vi "Teleop.vi"(10 "Match Info":T1={"Autonomous Elapsed Seconds"=0.0, "TeleOp Elapsed Seconds"=0.0, "Disabled Elapsed Seconds"=0.0, "Visited Autonomous"=FALSE, "Visited TeleOp"=FALSE, "Visited Disabled"=FALSE, "Autonomous Settings"={"Autonomous Style"=enum."Independent", "VI Refnum"=refnum}}, 11 "Call Context":T2) -> ()   [LabVIEW 2012]
doc: "This VI is called for each TeleOp packet received from the DS where the robot is not disabled. It is often used to read from the joysticks and update I/O or to update setpoints for timed control loops. It should complete and return within 20 milliseconds or it may miss DS packets."
uses:
  <vilib>/Rock Robotics/WPI/DriverStation/WPI_DriverStationDerivedRobotMode.ctl
  <vilib>/Rock Robotics/WPI/DriverStation/WPI_DriverStationMatch Info.ctl
  Sidestep Globals.vi
  Robot Global Data.vi
  <vilib>/Rock Robotics/Network Tables/SD Write Number.vi
  <vilib>/Rock Robotics/Network Tables/SD Write String.vi
  <vilib>/Rock Robotics/Network Tables/SD Write Boolean.vi
panel:
  in  "Hotkey Timer":dbl
  in  "Hotkey Step":i16
  out "Hotkey Running?":bool
  in  "Current Hotkey":string
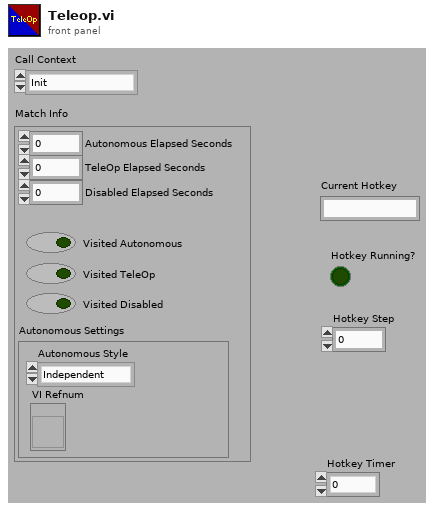
[diagram p1: front panel]
types:
  T1 = typedef "WPI_DriverStationMatch Info.ctl" = cluster{"Autonomous Elapsed Seconds":dbl, "TeleOp Elapsed Seconds":dbl, "Disabled Elapsed Seconds":dbl, "Visited Autonomous":bool, "Visited TeleOp":bool, "Visited Disabled":bool, "Autonomous Settings":cluster{"Autonomous Style":enum16{"Iterative", "Independent"}, "VI Refnum":refnum<vi>}}
  T2 = typedef "WPI_DriverStationDerivedRobotMode.ctl" = enum16{"Init", "Execute", "Stop"}
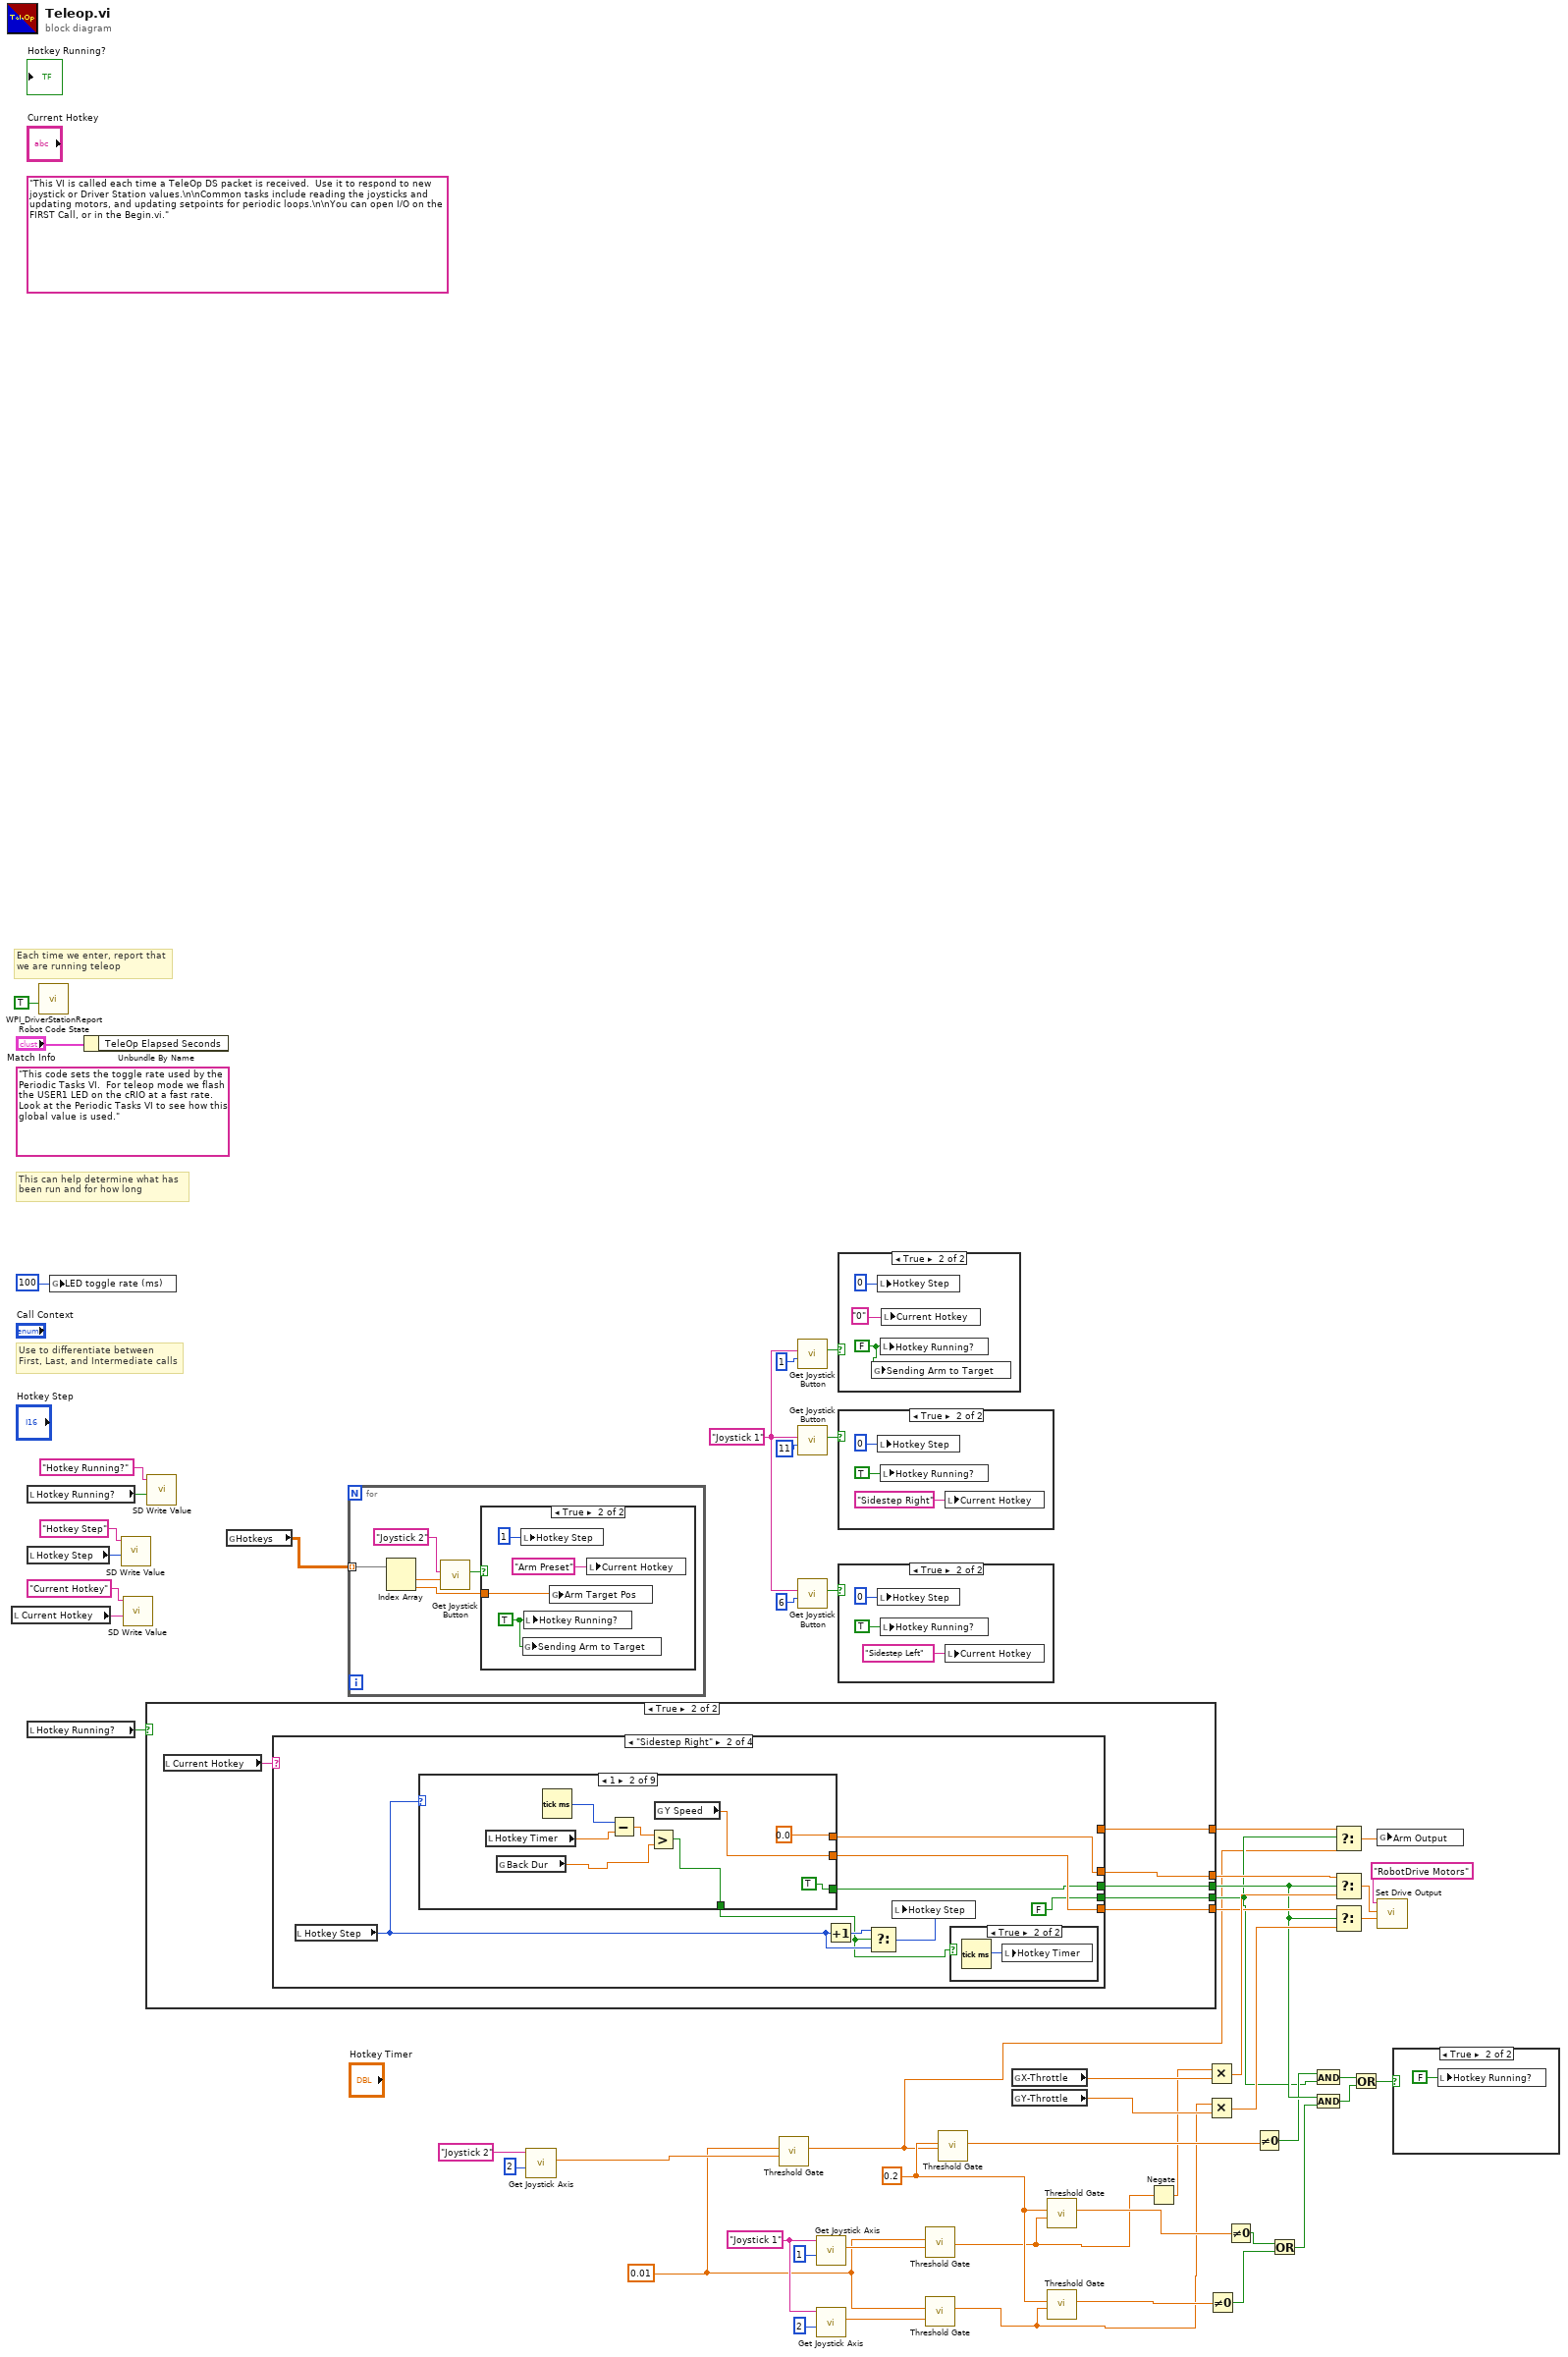
[diagram p0: block diagram]
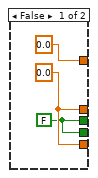
[diagram p5: hidden frame]
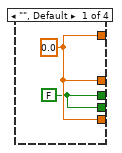
[diagram p6: hidden frame]
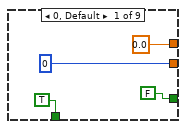
[diagram p8: hidden frame]
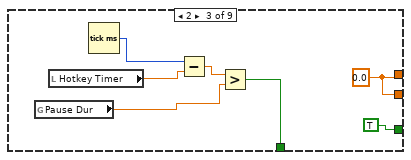
[diagram p9: hidden frame]
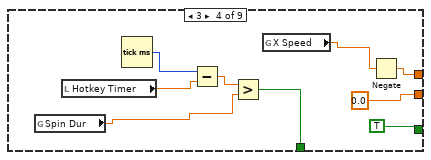
[diagram p10: hidden frame]
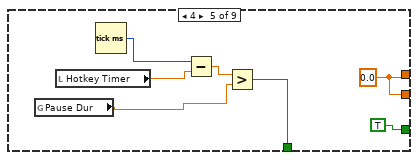
[diagram p11: hidden frame]
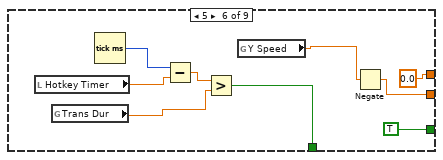
[diagram p12: hidden frame]
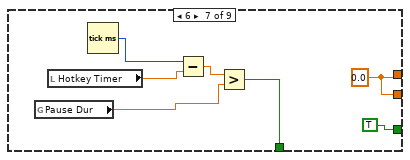
[diagram p13: hidden frame]
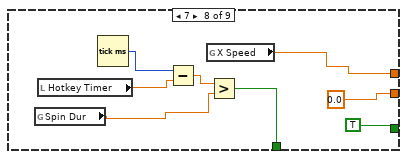
[diagram p14: hidden frame]
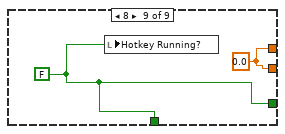
[diagram p15: hidden frame]
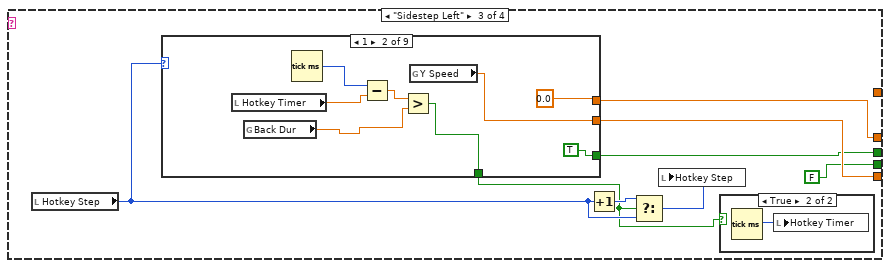
[diagram p16: hidden frame]
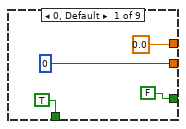
[diagram p18: hidden frame]
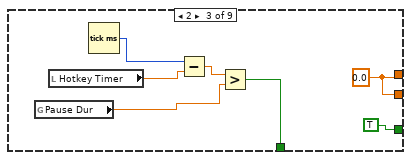
[diagram p19: hidden frame]
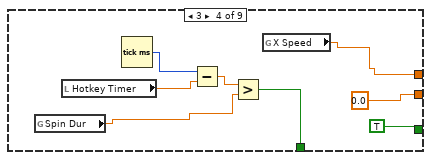
[diagram p20: hidden frame]
diagram:
  w9 = "Joystick 1"
  w30 = 0.2
  w48 = "Joystick 1"
  w13 = 0.01
  (unwired) "This code sets the toggle rate used by the Periodic Tasks VI.  For teleop mode we flash the USER1 LED on the cRIO at a fast rate.  Look at the Periodic Tasks VI to see how this global value is used."
  (unwired) "This VI is called each time a TeleOp DS packet is received.  Use it to respond to new joystick or Driver Station values.\n\nCommon tasks include reading the joysticks and updating motors, and updating setpoints for periodic loops.\n\nYou can open I/O on the FIRST Call, or in the Begin.vi."
  # "Each time we enter, report that\nwe are running teleop"
  # "Use to differentiate between\nFirst, Last, and Intermediate calls"
  # "This can help determine what has\nbeen run and for how long"
  n1 = local read "Current Hotkey"() -> (w27:string)
  n2 = local read "Hotkey Running?"() -> (w29:bool)
  n3 = local read "Hotkey Step"() -> (w28:i16)
  n4 = local read "Hotkey Running?"() -> (w40:bool)
  n5 = call <vilib>:"WPI_DriverStationReport Robot Code State.vi"("TeleOp"=TRUE ("Autonomous")) -> ()  [unwired: 10 in, 1 out]
  n6 = global write "Robot Global Data.vi" "LED toggle rate (ms)"(u32 100 ("LED ms toggle rate")) -> ()
  n7 = Unbundle By Name("Match Info") -> ()  [unwired: 1 out]
  n8 = call-poly <vilib>:"SD Write Value.vi"("Numeric"=w28, "Name"="Hotkey Step") -> ()  [unwired: 8 in, 2 out]
  n9 = call-poly <vilib>:"SD Write Value.vi"("String"=w27, "Name"="Current Hotkey") -> ()  [unwired: 8 in, 2 out]
  n10 = case shown="True" w40 {
    tunnel: [0.0 w63] -> w39
    tunnel: [w56 w62] -> w18
    tunnel: [w57 w60] -> w34
    tunnel: [w57 w61] -> w31
    tunnel: [w56 w59] -> w20
    frame False {
      w57 = 0.0
      w56 = FALSE
    }
    frame True {
      n11 = local read "Current Hotkey"() -> (w64:string)
      n12 = case shown="\"Sidestep Right\"" w64 {
        tunnel: [w66 _ _ w210] -> w63
        tunnel: [w65 FALSE FALSE w209] -> w62
        tunnel: [w66 w71 w141 w208] -> w61
        tunnel: [w66 w67 w137 w208] -> w60
        tunnel: [w65 w70 w140 FALSE] -> w59
        frame "", Default {
          w65 = FALSE
          w66 = 0.0
        }
        frame "Sidestep Right" {
          n13 = local read "Hotkey Step"() -> (w72:i16)
          n14 = case shown="1" w72 {
            tunnel: [TRUE w83 w90 w100 w106 w116 w122 w131 w136] -> w68
            tunnel: [0 w80 w94 0.0 w110 w111 w126 0.0 w135] -> w71
            tunnel: [FALSE TRUE TRUE TRUE TRUE TRUE TRUE TRUE w136] -> w70
            tunnel: [0.0 0.0 w94 w97 w110 0.0 w126 w127 w135] -> w67
            frame 0, Default {
            }
            frame 1 {
              n15 = local read "Hotkey Timer"() -> (w85:dbl)
              n16 = global read "Sidestep Globals.vi" "Back Dur"() -> (w81:dbl)
              n17 = Tick Count (ms)() -> (millisecond timer value=w86:u32)
              n18 = Subtract(x=w86, y=w85) -> (x-y=w84:dbl)
              n19 = Greater?(x=w84, y=w81) -> (0:w83:bool)
              n20 = global read "Sidestep Globals.vi" "Y Speed"() -> (w80:dbl)
            }
            frame 2 {
              w94 = 0.0
              n21 = global read "Sidestep Globals.vi" "Pause Dur"() -> (w88:dbl)
              n22 = local read "Hotkey Timer"() -> (w93:dbl)
              n23 = Tick Count (ms)() -> (millisecond timer value=w91:u32)
              n24 = Subtract(x=w91, y=w93) -> (x-y=w92:dbl)
              n25 = Greater?(x=w92, y=w88) -> (0:w90:bool)
            }
            frame 3 {
              n26 = global read "Sidestep Globals.vi" "Spin Dur"() -> (w96:dbl)
              n27 = local read "Hotkey Timer"() -> (w103:dbl)
              n28 = Tick Count (ms)() -> (millisecond timer value=w101:u32)
              n29 = Subtract(x=w101, y=w103) -> (x-y=w102:dbl)
              n30 = Greater?(x=w102, y=w96) -> (0:w100:bool)
              n31 = global read "Sidestep Globals.vi" "X Speed"() -> (w95:dbl)
              n32 = Negate(x=w95) -> (-x=w97:dbl)
            }
            frame 4 {
              w110 = 0.0
              n33 = global read "Sidestep Globals.vi" "Pause Dur"() -> (w104:dbl)
              n34 = local read "Hotkey Timer"() -> (w109:dbl)
              n35 = Tick Count (ms)() -> (millisecond timer value=w107:u32)
              n36 = Subtract(x=w107, y=w109) -> (x-y=w108:dbl)
              n37 = Greater?(x=w108, y=w104) -> (0:w106:bool)
            }
            frame 5 {
              n38 = local read "Hotkey Timer"() -> (w118:dbl)
              n39 = global read "Sidestep Globals.vi" "Trans Dur"() -> (w113:dbl)
              n40 = Tick Count (ms)() -> (millisecond timer value=w119:u32)
              n41 = Subtract(x=w119, y=w118) -> (x-y=w117:dbl)
              n42 = Greater?(x=w117, y=w113) -> (0:w116:bool)
              n43 = global read "Sidestep Globals.vi" "Y Speed"() -> (w112:dbl)
              n44 = Negate(x=w112) -> (-x=w111:dbl)
            }
            frame 6 {
              w126 = 0.0
              n45 = global read "Sidestep Globals.vi" "Pause Dur"() -> (w120:dbl)
              n46 = local read "Hotkey Timer"() -> (w125:dbl)
              n47 = Tick Count (ms)() -> (millisecond timer value=w123:u32)
              n48 = Subtract(x=w123, y=w125) -> (x-y=w124:dbl)
              n49 = Greater?(x=w124, y=w120) -> (0:w122:bool)
            }
            frame 7 {
              n50 = global read "Sidestep Globals.vi" "Spin Dur"() -> (w128:dbl)
              n51 = local read "Hotkey Timer"() -> (w134:dbl)
              n52 = Tick Count (ms)() -> (millisecond timer value=w132:u32)
              n53 = Subtract(x=w132, y=w134) -> (x-y=w133:dbl)
              n54 = global read "Sidestep Globals.vi" "X Speed"() -> (w127:dbl)
              n55 = Greater?(x=w133, y=w128) -> (0:w131:bool)
            }
            frame 8 {
              w135 = 0.0
              w136 = FALSE
              n56 = local write "Hotkey Running?"(w136) -> ()
            }
          }
          n57 = Increment(x=w72) -> (x+1=w74:i16)
          n58 = Select(t=w74, s=w68, f=w72) -> (s? t:f=w73:i16)
          n59 = local write "Hotkey Step"(w73) -> ()
          n60 = case shown="True" w68 {
            frame False {
            }
            frame True {
              n61 = Tick Count (ms)() -> (millisecond timer value=w75:u32)
              n62 = local write "Hotkey Timer"(w75) -> ()
            }
          }
        }
        frame "Sidestep Left" {
          n63 = local read "Hotkey Step"() -> (w142:i16)
          n64 = case shown="1" w142 {
            tunnel: [TRUE w153 w160 w169 w175 w185 w191 w201 w206] -> w138
            tunnel: [0 w150 w164 0.0 w179 w181 w195 0.0 w205] -> w141
            tunnel: [FALSE TRUE TRUE TRUE TRUE TRUE TRUE TRUE w206] -> w140
            tunnel: [0.0 0.0 w164 w165 w179 0.0 w195 w196 w205] -> w137
            frame 0, Default {
            }
            frame 1 {
              n65 = local read "Hotkey Timer"() -> (w155:dbl)
              n66 = global read "Sidestep Globals.vi" "Back Dur"() -> (w151:dbl)
              n67 = Tick Count (ms)() -> (millisecond timer value=w156:u32)
              n68 = Subtract(x=w156, y=w155) -> (x-y=w154:dbl)
              n69 = Greater?(x=w154, y=w151) -> (0:w153:bool)
              n70 = global read "Sidestep Globals.vi" "Y Speed"() -> (w150:dbl)
            }
            frame 2 {
              w164 = 0.0
              n71 = global read "Sidestep Globals.vi" "Pause Dur"() -> (w158:dbl)
              n72 = local read "Hotkey Timer"() -> (w163:dbl)
              n73 = Tick Count (ms)() -> (millisecond timer value=w161:u32)
              n74 = Subtract(x=w161, y=w163) -> (x-y=w162:dbl)
              n75 = Greater?(x=w162, y=w158) -> (0:w160:bool)
            }
            frame 3 {
              n76 = global read "Sidestep Globals.vi" "Spin Dur"() -> (w166:dbl)
              n77 = local read "Hotkey Timer"() -> (w172:dbl)
              n78 = Tick Count (ms)() -> (millisecond timer value=w170:u32)
              n79 = Subtract(x=w170, y=w172) -> (x-y=w171:dbl)
              n80 = Greater?(x=w171, y=w166) -> (0:w169:bool)
              n81 = global read "Sidestep Globals.vi" "X Speed"() -> (w165:dbl)
            }
            frame 4 {
              w179 = 0.0
              n82 = global read "Sidestep Globals.vi" "Pause Dur"() -> (w173:dbl)
              n83 = local read "Hotkey Timer"() -> (w178:dbl)
              n84 = Tick Count (ms)() -> (millisecond timer value=w176:u32)
              n85 = Subtract(x=w176, y=w178) -> (x-y=w177:dbl)
              n86 = Greater?(x=w177, y=w173) -> (0:w175:bool)
            }
            frame 5 {
              n87 = local read "Hotkey Timer"() -> (w187:dbl)
              n88 = global read "Sidestep Globals.vi" "Trans Dur"() -> (w182:dbl)
              n89 = Tick Count (ms)() -> (millisecond timer value=w188:u32)
              n90 = Subtract(x=w188, y=w187) -> (x-y=w186:dbl)
              n91 = Greater?(x=w186, y=w182) -> (0:w185:bool)
              n92 = global read "Sidestep Globals.vi" "Y Speed"() -> (w180:dbl)
              n93 = Negate(x=w180) -> (-x=w181:dbl)
            }
            frame 6 {
              w195 = 0.0
              n94 = global read "Sidestep Globals.vi" "Pause Dur"() -> (w189:dbl)
              n95 = local read "Hotkey Timer"() -> (w194:dbl)
              n96 = Tick Count (ms)() -> (millisecond timer value=w192:u32)
              n97 = Subtract(x=w192, y=w194) -> (x-y=w193:dbl)
              n98 = Greater?(x=w193, y=w189) -> (0:w191:bool)
            }
            frame 7 {
              n99 = global read "Sidestep Globals.vi" "Spin Dur"() -> (w199:dbl)
              n100 = local read "Hotkey Timer"() -> (w204:dbl)
              n101 = Tick Count (ms)() -> (millisecond timer value=w202:u32)
              n102 = Subtract(x=w202, y=w204) -> (x-y=w203:dbl)
              n103 = global read "Sidestep Globals.vi" "X Speed"() -> (w197:dbl)
              n104 = Greater?(x=w203, y=w199) -> (0:w201:bool)
              n105 = Negate(x=w197) -> (-x=w196:dbl)
            }
            frame 8 {
              w205 = 0.0
              w206 = FALSE
              n106 = local write "Hotkey Running?"(w206) -> ()
            }
          }
          n107 = Increment(x=w142) -> (x+1=w144:i16)
          n108 = Select(t=w144, s=w138, f=w142) -> (s? t:f=w143:i16)
          n109 = local write "Hotkey Step"(w143) -> ()
          n110 = case shown="True" w138 {
            frame False {
            }
            frame True {
              n111 = Tick Count (ms)() -> (millisecond timer value=w145:u32)
              n112 = local write "Hotkey Timer"(w145) -> ()
            }
          }
        }
        frame "Arm Preset" {
          w208 = 0.0
          n113 = local read "Hotkey Step"() -> (w213:i16)
          n114 = case shown="2" w213 {
            tunnel: [w215 w218] -> w214
            tunnel: [_ 0.0] -> w210
            tunnel: [FALSE w218] -> w209
            frame 1, Default {
              n115 = global read "Robot Global Data.vi" "Sending Arm to Target"() -> (w217:bool)
              n116 = Not(x=w217) -> (.not. x?=w215:bool)
            }
            frame 2 {
              w218 = FALSE
            }
          }
          n117 = Increment(x=w213) -> (x+1=w212:i16)
          n118 = Select(t=w212, s=w214, f=w213) -> (s? t:f=w211:i16)
          n119 = local write "Hotkey Step"(w211) -> ()
        }
      }
    }
  }
  n120 = call-poly <vilib>:"SD Write Value.vi"("Boolean"=w29, "Name"="Hotkey Running?") -> ()  [unwired: 8 in, 2 out]
  n121 = global read "Robot Global Data.vi" "Hotkeys"() -> (w52:dbl[][])
  n122 = for {
    tunnel: w52 -> [w223] mode=indexing
    n123 = Index Array(array=w223) -> (element #1=w222:dbl, element #2=w220:dbl)  [unwired: 2 in]
    n124 = call "Get Joystick Button.vi"("Button #"=w222, "Joystick RefNum"="Joystick 2") -> ("Value"=w221:bool)  [unwired: 9 in]
    n125 = case shown="True" w221 {
      tunnel: w220 -> [_ w226]
      frame False {
      }
      frame True {
        w225 = TRUE
        n126 = local write "Hotkey Step"(1) -> ()
        n127 = global write "Robot Global Data.vi" "Sending Arm to Target"(w225) -> ()
        n128 = local write "Hotkey Running?"(w225) -> ()
        n129 = global write "Robot Global Data.vi" "Arm Target Pos"(w226) -> ()
        n130 = local write "Current Hotkey"("Arm Preset") -> ()
      }
    }
  }
  n131 = call "Get Joystick Axis.vi"("Axis"=2, "Joystic Ref"="Joystick 2") -> ("Value"=w49:dbl)  [unwired: 9 in]
  n132 = call "Threshold Gate.vi"("Value"=w49, "Threshold"=w13) -> ("Output"=w3:dbl)  [unwired: 9 in]
  n133 = call "Get Joystick Button.vi"("Button #"=1, "Joystick RefNum"=w9) -> ("Value"=w10:bool)  [unwired: 9 in]
  n134 = call "Get Joystick Button.vi"("Button #"=11, "Joystick RefNum"=w9) -> ("Value"=w12:bool)  [unwired: 9 in]
  n135 = call "Get Joystick Button.vi"("Button #"=6, "Joystick RefNum"=w9) -> ("Value"=w11:bool)  [unwired: 9 in]
  n136 = call "Get Joystick Axis.vi"("Axis"=1, "Joystic Ref"=w48) -> ("Value"=w15:dbl)  [unwired: 9 in]
  n137 = call "Get Joystick Axis.vi"("Axis"=2, "Joystic Ref"=w48) -> ("Value"=w14:dbl)  [unwired: 9 in]
  n138 = case shown="True" w10 {
    frame False {
    }
    frame True {
      w229 = FALSE
      n139 = global write "Robot Global Data.vi" "Sending Arm to Target"(w229) -> ()
      n140 = local write "Hotkey Step"(0) -> ()
      n141 = local write "Hotkey Running?"(w229) -> ()
      n142 = local write "Current Hotkey"("0") -> ()
    }
  }
  n143 = case shown="True" w12 {
    frame False {
    }
    frame True {
      n144 = local write "Hotkey Step"(0) -> ()
      n145 = local write "Hotkey Running?"(TRUE) -> ()
      n146 = local write "Current Hotkey"("Sidestep Right") -> ()
    }
  }
  n147 = case shown="True" w11 {
    frame False {
    }
    frame True {
      n148 = local write "Hotkey Step"(0) -> ()
      n149 = local write "Hotkey Running?"(TRUE) -> ()
      n150 = local write "Current Hotkey"("Sidestep Left") -> ()
    }
  }
  n151 = call "Threshold Gate.vi"("Value"=w15, "Threshold"=w13) -> ("Output"=w2:dbl)  [unwired: 9 in]
  n152 = call "Threshold Gate.vi"("Value"=w14, "Threshold"=w13) -> ("Output"=w1:dbl)  [unwired: 9 in]
  n153 = call "Threshold Gate.vi"("Value"=w3, "Threshold"=w30) -> ("Output"=w41:dbl)  [unwired: 9 in]
  n154 = global read "Robot Global Data.vi" "X-Throttle"() -> (w44:dbl)
  n155 = global read "Robot Global Data.vi" "Y-Throttle"() -> (w43:dbl)
  n156 = call "Threshold Gate.vi"("Value"=w2, "Threshold"=w30) -> ("Output"=w5:dbl)  [unwired: 9 in]
  n157 = call "Threshold Gate.vi"("Value"=w1, "Threshold"=w30) -> ("Output"=w37:dbl)  [unwired: 9 in]
  n158 = Negate(x=w2) -> (-x=w38:dbl)
  n159 = Multiply(x=w38, y=w44) -> (x*y=w36:dbl)
  n160 = Multiply(x=w1, y=w43) -> (x*y=w33:dbl)
  n161 = Not Equal To 0?(x=w37) -> (x != 0?=w23:bool)
  n162 = Not Equal To 0?(x=w5) -> (x != 0?=w22:bool)
  n163 = Not Equal To 0?(x=w41) -> (x != 0?=w19:bool)
  n164 = Or(x=w22, y=w23) -> (x .or. y?=w21:bool)
  n165 = And(x=w19, y=w18) -> (x .and. y?=w4:bool)
  n166 = And(x=w20, y=w21) -> (x .and. y?=w16:bool)
  n167 = Select(t=w39, s=w18, f=w3) -> (s? t:f=w42:dbl)
  n168 = Select(t=w34, s=w20, f=w36) -> (s? t:f=w35:dbl)
  n169 = Select(t=w31, s=w20, f=w33) -> (s? t:f=w32:dbl)
  n170 = Or(x=w4, y=w16) -> (x .or. y?=w17:bool)
  n171 = global write "Robot Global Data.vi" "Arm Output"(w42) -> ()
  n172 = call "Set Drive Output.vi"("Y axis"=w32, "X axis"=w35, "Drive RefNum"="RobotDrive Motors" ("Name")) -> ()  [unwired: 7 in]
  n173 = case shown="True" w17 {
    frame False {
    }
    frame True {
      n174 = local write "Hotkey Running?"(FALSE) -> ()
    }
  }
